vi "DragDropMoveCopyIsAcceptable.vi"(4 "Copy?":bool, 5 "element":cluster{"Parent":i32, "Child":i32}, 6 "Insert Index":i32, 7 "Allowed Parent Child":set{cluster{"Parent":i32, "Child":i32}}(c389), 8 "error in (no error)":errorcluster, 9 "Data Tag":string, 10 "Parent Tag":string, 11 "TreeControl in":refnum<vi>) -> (0 "error out":errorcluster, 1 "Acceptable":bool, 3 "TreeControl out":refnum<vi>)   [LabVIEW 2020, in "TreeControlLib.lvlib"]
uses:
  TreeControlLib.lvlib
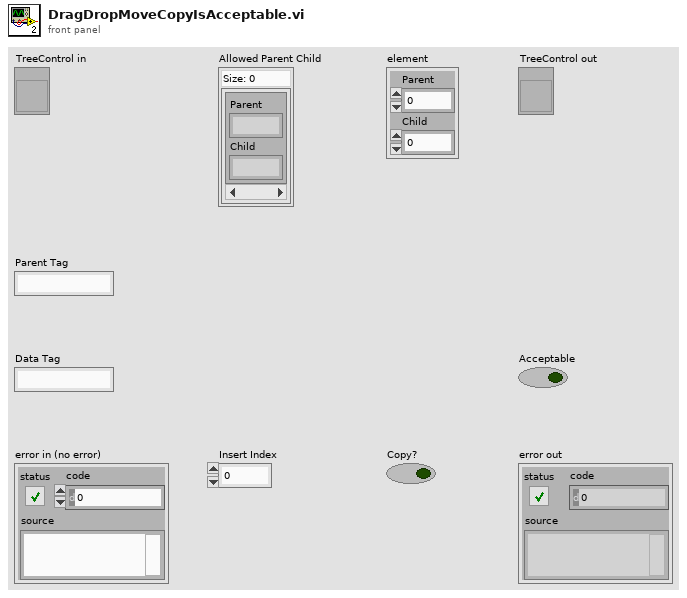
[diagram p1: front panel]
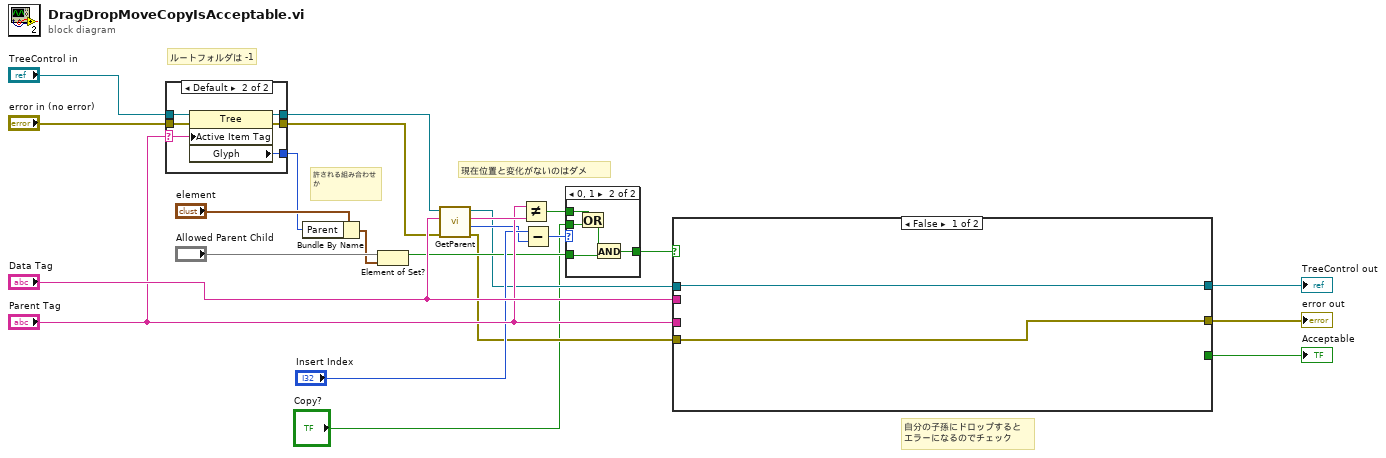
[diagram p0: block diagram]
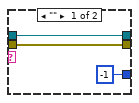
[diagram p3: hidden frame]
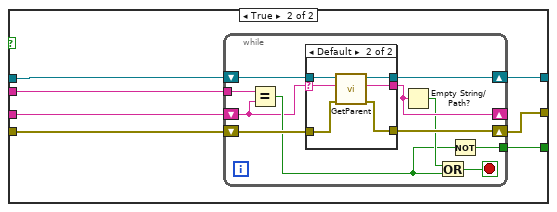
[diagram p4: hidden frame]
diagram:
  # "現在位置と変化がないのはダメ"
  # "ルートフォルダは -1"
  # "許される組み合わせか"
  # "自分の子孫にドロップすると\nエラーになるのでチェック"
  n1 = case shown="Default" "Parent Tag" {
    selector: "Parent Tag" -> [_ w27]
    tunnel: "TreeControl in" -> [w25 w32]
    tunnel: [w24 w31] -> w4
    tunnel: [w25 w30] -> w13
    tunnel: "error in (no error)" -> [w24 w29]
    tunnel: [-1 ("Glyph") w28] -> w15
    frame "" {
    }
    frame Default {
      n2 = property class="Tree"(reference=w32, error in=w29, "Active Item Tag"=w27) -> (reference out=w30:refnum<vi>, error out=w31:errorcluster, "Glyph"=w28:i32)
    }
  }
  n3 = Bundle By Name(cluster="element", "Parent"=w15) -> (w16:cluster{"Parent":i32, "Child":i32})
  n4 = Element of Set?(10:w16, 11:"Allowed Parent Child") -> (3:w7:bool)
  n5 = call "GetParent.vi"("error in (no error)"=w4, "Tag"="Data Tag", "TreeControl in"=w13) -> ("error out"=w3:errorcluster, "Child Index"=w9:i32, "Parent Tag"=w14:string, "TreeControl out"=w2:refnum<vi>)  [unwired: 5 in]
  n6 = Not Equal?(x="Parent Tag", y=w14) -> (x != y?=w5:bool)
  n7 = Subtract(x="Insert Index", y=w9) -> (x-y=w8:i32)
  n8 = case shown="0, 1" w8 {
    tunnel: w7 -> [w33 w37]
    tunnel: [w33 w38] -> w6
    tunnel: w5 -> [_ w36]
    tunnel: "Copy?" -> [_ w34]
    frame Default {
    }
    frame 0, 1 {
      n9 = Or(x=w36, y=w34) -> (x .or. y?=w35:bool)
      n10 = And(x=w35, y=w37) -> (x .and. y?=w38:bool)
    }
  }
  n11 = case shown="False" w6 {
    tunnel: "Data Tag" -> [_ w47]
    tunnel: "Parent Tag" -> [_ w46]
    tunnel: [w40 w45] -> w20
    tunnel: w3 -> [w40 w44]
    tunnel: [_ w43] -> w18
    tunnel: [w39 w42] -> w19
    tunnel: w2 -> [w39 w41]
    frame False {
    }
    frame True {
      n12 = while {
        tunnel: w47 -> [w58]
        shift-right: [w54] -> _
        shift-left: w46 -> [w48]
        shift-right: [w55] -> w45
        shift-left: w44 -> [w56]
        tunnel: [w50] -> w43
        shift-right: [w49] -> w42
        shift-left: w41 -> [w57]
        stop <- w52 stop-if-true
        n13 = Equal?(x=w58, y=w48) -> (x = y?=w51:bool)
        n14 = case shown="Default" w48 {
          selector: w48 -> [_ w61]
          tunnel: w57 -> [w60 w66]
          tunnel: w56 -> [w59 w65]
          tunnel: [w59 w64] -> w55
          tunnel: [_ w63] -> w54
          tunnel: [w60 w62] -> w49
          frame "" {
          }
          frame Default {
            n15 = call "GetParent.vi"("error in (no error)"=w65, "Tag"=w61, "TreeControl in"=w66) -> ("error out"=w64:errorcluster, "Parent Tag"=w63:string, "TreeControl out"=w62:refnum<vi>)  [unwired: 5 in, 1 out]
          }
        }
        n16 = Empty String/Path?(string/path=w54) -> (empty?=w53:bool)
        n17 = Or(x=w53, y=w51) -> (x .or. y?=w52:bool)
        n18 = Not(x=w51) -> (.not. x?=w50:bool)
      }
    }
  }
  "error out" <- w20
  "TreeControl out" <- w19
  "Acceptable" <- w18
